vi "Calibrate Gripper.vi"(2 "node":string, 3 "Side":T1, 6 "error in":errorcluster) -> (5 "error out":errorcluster)   [LabVIEW 2012]
doc: "Calibrate the left or right gripper"
uses:
  <userlib>/rosforlv/ROS/Code/SubVIs/BaxterSide.ctl
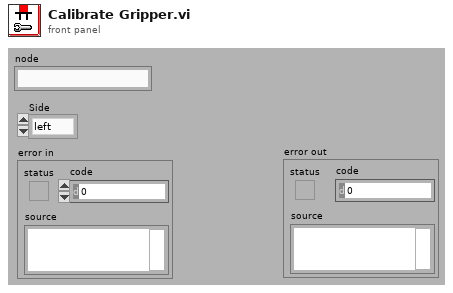
[diagram p1: front panel]
types:
  T1 = typedef "BaxterSide.ctl" = enum16{"left", "right"}
  T2 = enum16{"no_op", "set", "configure", "reboot", "reset", "calibrate", "clear_calibration", "prepare_to_grip", "grip", "release", "go", "stop"}
  T3 = typedef "TopicDef.ctl" = cluster{"Topic":string, "Type":string, "Action":T4, "Update (ms)":u16, "write queue":u16}
  T4 = typedef "_ROSDirection.ctl" = enum16{"Node", "Publisher", "Subscriber", "Service Client"}
  T5 = typedef "_ROSControl.ctl" = cluster{"topic port":u16, "Node":string, "topic":string, "type":string, "node port":u32, "error ":errorcluster, "Direction":T4, "APIs":string[], "Update (ms)":u16, "write queue":u16}
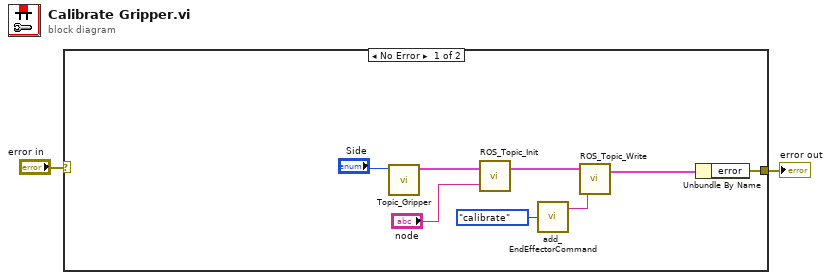
[diagram p0: block diagram]
diagram:
  n1 = case shown="No Error" "error in" {
    selector: "error in" -> [_ w11]
    tunnel: [w8 w11] -> w2
    frame No Error {
      n2 = call <userlib>:"Topic_Gripper.vi"("Side"="Side") -> ("Definitions"=w5:T3)  [unwired: 10 in]
      n3 = call <userlib>:"ROS_Topic_Init.vi"("node"="node", "Definitions"=w5) -> ("ROS out"=w10:T5)  [unwired: 1 in]
      n4 = call <userlib>:"add_EndEffectorCommand.vi"("Commands"=T2."calibrate") -> ("msg out"=w4:string)  [unwired: 4 in]
      n5 = call <userlib>:"ROS_Topic_Write.vi"("Msg in"=w4, "ROS in"=w10) -> ("ROS out"=w9:T5)  [unwired: 2 in]
      n6 = Unbundle By Name(w9) -> ("error"=w8:errorcluster)
    }
    frame Error {
    }
  }
  "error out" <- w2
